vi "Wire Measurement Wrapper.vi"(0 "vi reference":refnum<vi>, 5 "SubVI in":refnum<vi>[](array[refnum]), 7 "Terminal":refnum<vi>, 11 "error in (no error)":errorcluster) -> (15 "error out":errorcluster)   [LabVIEW 2021, in "Migrator.lvlib"]
uses:
  Migrator.lvlib
  Migrator Reusables/Migrator Reusables.lvlib
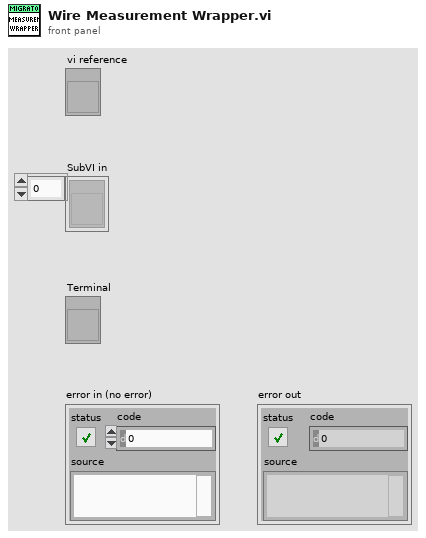
[diagram p1: front panel]
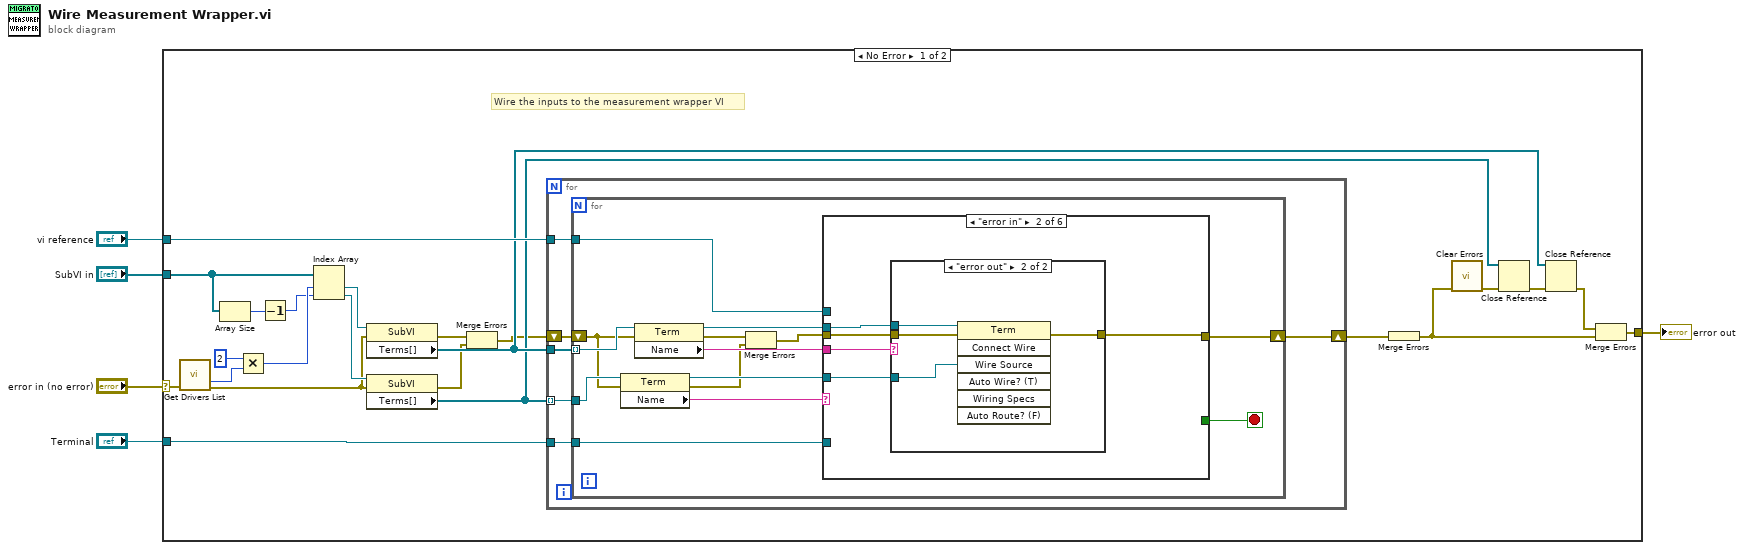
[diagram p0: block diagram]
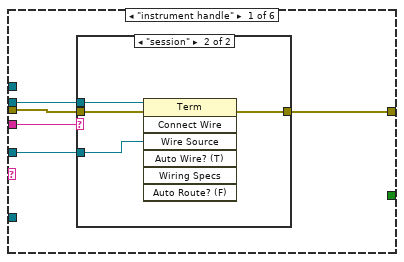
[diagram p2: hidden frame]
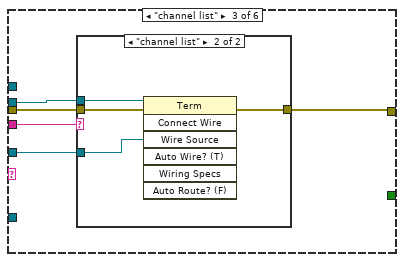
[diagram p5: hidden frame]
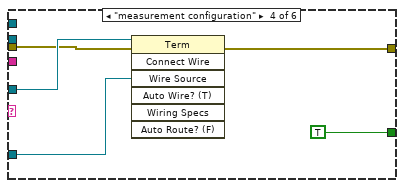
[diagram p7: hidden frame]
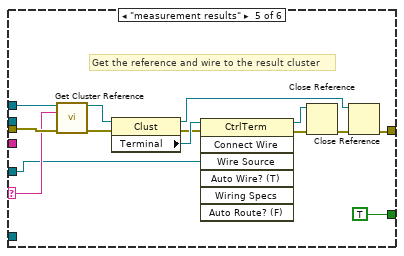
[diagram p8: hidden frame]
diagram:
  n1 = case shown="No Error" "error in (no error)" {
    selector: "error in (no error)" -> [w15 w99]
    tunnel: "vi reference" -> [w24 _]
    tunnel: [w18 w99] -> w4
    tunnel: "Terminal" -> [w16 _]
    tunnel: "SubVI in" -> [w13 _]
    frame No Error {
      # "Wire the inputs to the measurement wrapper VI"
      n2 = call "Get Drivers List.vi"("error in (no error)"=w15) -> ("Removed Duplicates Size"=w9:i32, "error out"=w14:errorcluster)  [unwired: 9 in, 4 out]
      n3 = Array Size(array=w13) -> (size(s)=w12:i32)
      n4 = Multiply(x=2, y=w9) -> (x*y=w7:i32)
      n5 = Decrement(x=w12) -> (x-1=w6:i32)
      n6 = Index Array(array=w13, index #1=w7, index #2=w6) -> (element #1=w28:refnum<vi>, element #2=w27:refnum<vi>)
      n7 = property class="SubVI"(reference=w28, error in=w14) -> (error out=w26:errorcluster, "Terms[]"=w23:refnum<vi>[])  [unwired: 1 out]
      n8 = property class="SubVI"(reference=w27, error in=w14) -> (error out=w10:errorcluster, "Terms[]"=w22:refnum<vi>[])  [unwired: 1 out]
      n9 = Merge Errors(w26, w10) -> (w11:errorcluster)
      n10 = for {
        tunnel: w22 -> [w32] mode=indexing
        tunnel: w23 -> [w34]
        tunnel: w16 -> [w31]
        tunnel: w24 -> [w30]
        shift-right: [w29] -> w25
        shift-left: w11 -> [w33]
        n11 = for {
          tunnel: w34 -> [w48] mode=indexing
          tunnel: w32 -> [w47]
          tunnel: w31 -> [w44]
          tunnel: w30 -> [w39]
          shift-right: [w42] -> w29
          shift-left: w33 -> [w37]
          stop <- w38 stop-if-true
          n12 = property class="Term"(reference=w47, error in=w37) -> (reference out=w45:refnum<vi>, error out=w35:errorcluster, "Name"=w46:string)
          n13 = property class="Term"(reference=w48, error in=w37) -> (reference out=w40:refnum<vi>, error out=w43:errorcluster, "Name"=w41:string)
          n14 = Merge Errors(w43, w35) -> (w36:errorcluster)
          n15 = case shown="\"error in\"" w46 {
            selector: w46 -> [_ _ _ _ w96 _]
            tunnel: w45 -> [w51 w61 w71 w83 w92 _]
            tunnel: w44 -> [_ _ _ w81 _ _]
            tunnel: w36 -> [w52 w62 w72 w82 w97 w98]
            tunnel: [w49 w59 w69 w80 w87 w98] -> w42
            tunnel: w41 -> [w53 w63 w73 _ _ _]
            tunnel: w40 -> [w50 w60 w70 _ _ _]
            tunnel: w39 -> [_ _ _ _ w95 _]
            tunnel: [_ _ _ TRUE TRUE _] -> w38
            frame "instrument handle" {
              n16 = case shown="\"session\"" w53 {
                tunnel: w52 -> [w54 w58]
                tunnel: w51 -> [_ w57]
                tunnel: w50 -> [_ w56]
                tunnel: [w54 w55] -> w49
                frame Default {
                }
                frame "session" {
                  n17 = invoke class="Term" method="Connect Wire"(reference=w56, error in=w58, "Wire Source"=w57) -> (error out=w55:errorcluster)  [unwired: 4 in, 6 out]
                }
              }
            }
            frame "error in" {
              n18 = case shown="\"error out\"" w63 {
                tunnel: w62 -> [w64 w68]
                tunnel: w61 -> [_ w67]
                tunnel: w60 -> [_ w66]
                tunnel: [w64 w65] -> w59
                frame Default {
                }
                frame "error out" {
                  n19 = invoke class="Term" method="Connect Wire"(reference=w66, error in=w68, "Wire Source"=w67) -> (error out=w65:errorcluster)  [unwired: 4 in, 6 out]
                }
              }
            }
            frame "channel list" {
              n20 = case shown="\"channel list\"" w73 {
                tunnel: w72 -> [w74 w78]
                tunnel: w71 -> [_ w77]
                tunnel: w70 -> [_ w76]
                tunnel: [w74 w75] -> w69
                frame Default {
                }
                frame "channel list" {
                  n21 = invoke class="Term" method="Connect Wire"(reference=w76, error in=w78, "Wire Source"=w77) -> (error out=w75:errorcluster)  [unwired: 4 in, 6 out]
                }
              }
            }
            frame "measurement configuration" {
              n22 = invoke class="Term" method="Connect Wire"(reference=w83, error in=w82, "Wire Source"=w81) -> (error out=w80:errorcluster)  [unwired: 4 in, 6 out]
            }
            frame "measurement results" {
              # "Get the reference and wire to the result cluster"
              n23 = call "Get Cluster Reference.vi"("VI in"=w95, "name/order"=w96, "error in (no error)"=w97) -> ("Cluster out"=w88:refnum<vi>, "error out"=w94:errorcluster)  [unwired: 11 in]
              n24 = property class="Clust"(reference=w88, error in=w94) -> (reference out=w84:refnum<vi>, error out=w91:errorcluster, "Terminal"=w93:refnum<vi>)
              n25 = invoke class="CtrlTerm" method="Connect Wire"(reference=w93, error in=w91, "Wire Source"=w92) -> (reference out=w85:refnum<vi>, error out=w90:errorcluster)  [unwired: 4 in, 5 out]
              n26 = Close Reference(reference=w85, error in (no error)=w90) -> (error out=w89:errorcluster)
              n27 = Close Reference(reference=w84, error in (no error)=w89) -> (error out=w87:errorcluster)
            }
            frame Default {
            }
          }
        }
      }
      n28 = Merge Errors(w25) -> (w21:errorcluster)
      n29 = call <vilib>:"Clear Errors.vi"("error in (no error)"=w21) -> ("error out"=w20:errorcluster)  [unwired: 5 in, 1 out]
      n30 = Close Reference(reference=w22, error in (no error)=w20) -> (error out=w19:errorcluster)
      n31 = Close Reference(reference=w23, error in (no error)=w19) -> (error out=w17:errorcluster)
      n32 = Merge Errors(w17, w21) -> (w18:errorcluster)
    }
    frame Error {
    }
  }
  "error out" <- w4
